vi "Drivetrain Targeting.vi"() -> (3 "Drivetrain Center":dbl)   [LabVIEW 2012]
uses:
  Robot Global Data.vi
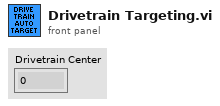
[diagram p1: front panel]
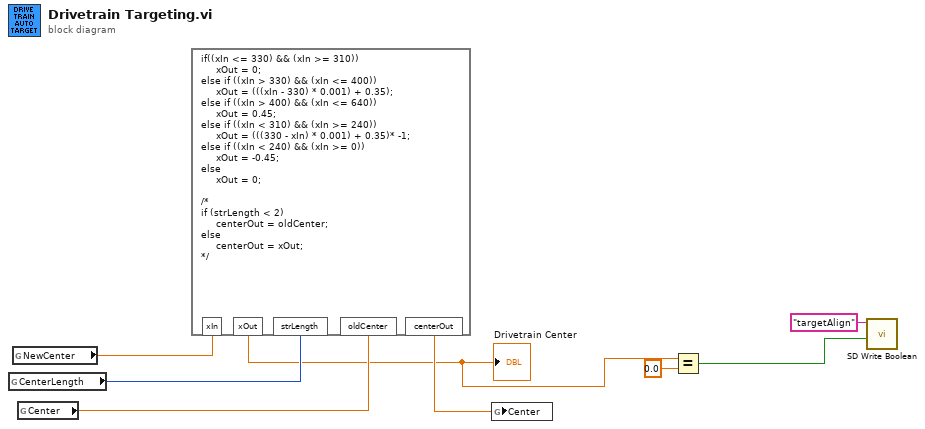
[diagram p0: block diagram]
diagram:
  n1 = global read "Robot Global Data.vi" "CenterLength"() -> (w5:i8)
  n2 = global read "Robot Global Data.vi" "NewCenter"() -> (w6:dbl)
  n3 = global read "Robot Global Data.vi" "Center"() -> (w8:dbl)
  n4 = formula code="if((xIn <= 330) && (xIn >= 310))\n     xOut = 0;\nelse if ((xIn > 330) && (xIn <= 400))\n     xOut = (((xIn - 330) * 0.001) + 0.35);\nelse if ((xIn > 400) && (xIn <= 640))\n     xOut = 0.45;\nelse if ((xIn < 310) && (xIn >= 240))\n     xOut = (((330 - xIn) * 0.001) + 0.35)* -1;\nelse if ((xIn < 240) && (xIn >= 0))\n     xOut = -0.45;\nelse\n     xOut = 0;\n\n/*\nif (strLength < 2) \n     centerOut = oldCenter;\nelse\n     centerOut = xOut;\n*/"("xIn"=w6, "oldCenter"=w8, "strLength"=w5) -> ("xOut"=w3:dbl, "centerOut"=w7:dbl)
  "Drivetrain Center" <- w3
  n5 = global write "Robot Global Data.vi" "Center"(w7) -> ()
  n6 = Equal?(x=w3, y=0.0) -> (x = y?=w1:bool)
  n7 = call <vilib>:"SD Write Boolean.vi"("Boolean"=w1, "Name"="targetAlign") -> ()  [unwired: 8 in, 2 out]
